vi "Auto Move Straight.vi"(7 "Target Distance":dbl=15.0 format="%#_13g", 8 "Error In":errorcluster, 11 "Refnum's In":T1) -> (0 "Error Out":errorcluster, 3 "Refnum's Out":T1)   [LabVIEW 2016]
uses:
  <vilib>/Rock Robotics/WPI/Utilities/WPI_GetSetVariantRefNum.vi
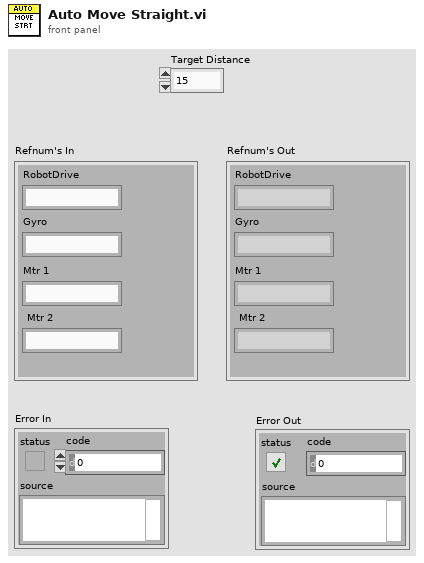
[diagram p1: front panel]
types:
  T1 = cluster{"RobotDrive":string, "Gyro":string, "Mtr 1":string, "Mtr 2":string}
  T2 = typedef "WPI_MotorControlDeviceRef.ctl" = cluster{"DeviceStatus":errorcluster, "Type":T3, "PWM":cluster{"PWM Channel":T4, "DeadBand":T5}, "CAN":cluster{"Device Number":u8, "SetOutput VI Ref":variant, "GetOutput VI Ref":variant, "Enable VI Ref":variant, "Disable VI Ref":variant, "Data":variant}, "Invert":bool}
  T3 = typedef "WPI_MotorControlType.ctl" = enum16{"PWM", "CAN"}
  T4 = typedef "FPGA_DIOPWMChannel.ctl" = enum8{"PWM 0", "PWM 1", "PWM 2", "PWM 3", "PWM 4", "PWM 5", "PWM 6", "PWM 7", "PWM 8", "PWM 9", "PWM MXP 0", "PWM MXP 1", "PWM MXP 2", "PWM MXP 3", "PWM MXP 4", "PWM MXP 5", "PWM MXP 6", "PWM MXP 7", "PWM MXP 8", "PWM MXP 9", "Invalid"}
  T5 = typedef "WPI_PWMDeadband.ctl" = cluster{"Name":string, "maxPositivePwm":i32, "minPositivePwm":i32, "centerPwm":i32, "maxNegativePwm":i32, "minNegativePwm":i32, "angularRange":u16}
  T6 = typedef "WPI_GyroDevRef.ctl" = cluster{"DevStatus":errorcluster, "Analog Channel":T7, "Offset":dbl, "Gain (VoltsPerDegree/Second)":dbl, "Gyro Type":enum16{"Analog", "XRS450"}, "Handle":i32, "SPI Bus":T8, "Device Found":bool, "Sample Rate":dbl, "Calibrate On Open":bool}
  T7 = typedef "FPGA_AIChannel.ctl" = enum8{"AI 0", "AI 1", "AI 2", "AI 3", "AI MXP 0", "AI MXP 1", "AI MXP 2", "AI MXP 3", "Invalid"}
  T8 = typedef "spi_bus.ctl" = enum16{"SPI On-Board, CS0", "SPI On-Board, CS1", "SPI On-Board, CS2", "SPI On-Board, CS3", "SPI MXP", "Invalid"}
  T9 = typedef "WPI_RobotDriveDevRef.ctl" = cluster{"DevStatus":errorcluster, "Motors[]":T2[], "Square Inputs":bool, "Max Output":dbl}
  T10 = typedef "WPI_CANTalonSRX_GlobalStatus.ctl" = cluster{"Applied Throttle":dbl, "Module Enabled":bool, "CAN Error":errorcluster, "Closed Loop Error":dbl, "Forward Limit Switch Closed":bool, "Reverse Limit Switch Closed":bool, "Sensor Position":dbl, "Sensor Velocity":dbl, "Current":dbl, "Sticky Fault - Over Temp":bool, "Sticky Fault - Under Voltage":bool, "Sticky Fault - Forward Limit":bool, "Sticky Fault - Reverse Limit":bool, "Sticky Fault - Forward Soft Limit":bool, "Sticky Fault - Reverse Soft Limit":bool, "Brake is Enabled":bool, "Encoder Position":dbl, "Encoder Velocity":dbl, "Encoder Index Count":dbl, "Encoder A Pin State":bool, "Encoder B Pin State":bool, "Encoder Index Pin State":bool, "Analog In":dbl, "Analog In Velocity":dbl, "Temperature (C)":dbl, "Battery Voltage":dbl, "Control 5 Is Supported":bool, "Current Profile Slot Select":dbl, "Pos Div 8":bool, "Vel Div 4":bool, "Pulse Width Position":i32, "Pulse Width Velocity":i32, "Pulse Width Rise To Rise (us)":i32, "Pulse Width Rise To Fall (us)":i32, "Mot Prof Active Is Under Run":bool, "Mot Prof Active Has Under Run":bool, "Mot Prof Active Is Last":bool, "Mot Prof Active Velocity Only":bool, "Mot Prof Active Is Valid":bool, "Mot Prof Buffer Is Full":bool, "Mot Prof Active Profile Slot Select":i32, "Mot Prof NextID":i32, "Mot Prof Count":i32, "Mot Prof Active Velocity":dbl, "Mot Prof Active Position":dbl, "Mot Prof Output Enable":i32}
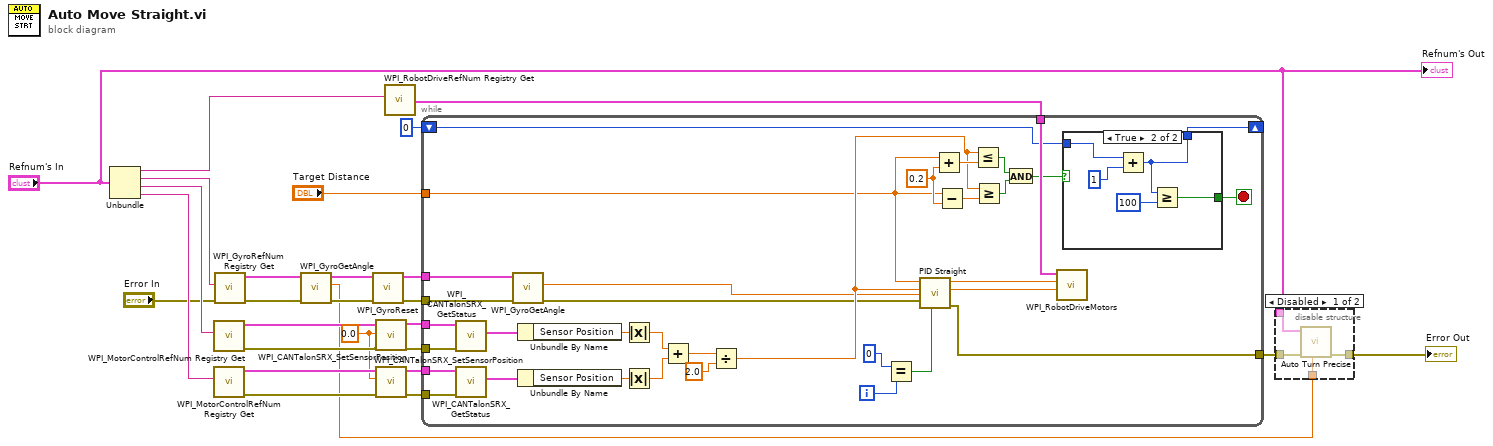
[diagram p0: block diagram]
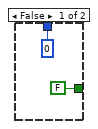
[diagram p3: hidden frame]
diagram:
  w16 = 0.0 ("New Sensor Position")
  n1 = Unbundle("Refnum's In") -> ("RobotDrive"=w11:string, "Gyro"=w10:string, "Mtr 1"=w9:string, "Mtr 2"=w8:string)
  n2 = call <vilib>:"WPI_MotorControlRefNum Registry Get.vi"("refnum name"=w9) -> ("error out"=w19:errorcluster, "MotorControlDevRef"=w20:T2)  [unwired: 9 in]
  n3 = call <vilib>:"WPI_MotorControlRefNum Registry Get.vi"("refnum name"=w8) -> ("error out"=w22:errorcluster, "MotorControlDevRef"=w21:T2)  [unwired: 9 in]
  n4 = call <vilib>:"WPI_GyroRefNum Registry Get.vi"("error in (no error)"="Error In", "refnum name"=w10) -> ("error out"=w1:errorcluster, "GyroDevRef"=w2:T6)  [unwired: 8 in]
  n5 = call <vilib>:"WPI_GyroGetAngle.vi"("error in"=w1, "GyroDevRef"=w2) -> ("error out"=w25:errorcluster, "Angle"=w3:dbl, "GyroDevRef"=w26:T6)  [unwired: 5 in, 2 out]
  n6 = call <vilib>:"WPI_GyroReset.vi"("error in"=w25, "GyroDevRef"=w26) -> ("error out"=w24:errorcluster, "GyroDevRef"=w23:T6)  [unwired: 8 in]
  n7 = call <vilib>:"WPI_CANTalonSRX_SetSensorPosition.vi"("error in (no error)"=w19, "New Sensor Position"=w16, "CAN Talon SRX Ref"=w20) -> ("error out"=w15:errorcluster, "CAN Talon SRX Ref"=w14:T2)  [unwired: 7 in]
  n8 = call <vilib>:"WPI_CANTalonSRX_SetSensorPosition.vi"("error in (no error)"=w22, "New Sensor Position"=w16, "CAN Talon SRX Ref"=w21) -> ("error out"=w17:errorcluster, "CAN Talon SRX Ref"=w18:T2)  [unwired: 7 in]
  n9 = call <vilib>:"WPI_RobotDriveRefNum Registry Get.vi"("refnum name"=w11) -> ("RobotDriveDevRef"=w12:T9)  [unwired: 9 in, 1 out]
  n10 = while {
    tunnel: w12 -> [w57]
    tunnel: w23 -> [w48]
    tunnel: w24 -> [w47]
    tunnel: w14 -> [w46]
    tunnel: w15 -> [w45]
    tunnel: w18 -> [w44]
    tunnel: w17 -> [w43]
    shift-right: [w35] -> _
    shift-left: 0 -> [w34]
    tunnel: "Target Distance" -> [w32]
    tunnel: [w29] -> w7
    i -> [w59]
    stop <- w28 stop-if-true
    w42 = 0.2 ("y")
    n11 = call <vilib>:"WPI_CANTalonSRX_GetStatus.vi"("error in (no error)"=w45, "CAN Talon SRX Ref"=w46) -> ("Talon SRX Status"=w49:T10)  [unwired: 7 in, 2 out]
    n12 = call <vilib>:"WPI_CANTalonSRX_GetStatus.vi"("error in (no error)"=w43, "CAN Talon SRX Ref"=w44) -> ("Talon SRX Status"=w50:T10)  [unwired: 7 in, 2 out]
    n13 = call <vilib>:"WPI_GyroGetAngle.vi"("error in"=w47, "GyroDevRef"=w48) -> ("error out"=w30:errorcluster, "Angle"=w33:dbl)  [unwired: 5 in, 3 out]
    n14 = Unbundle By Name(w49) -> ("Sensor Position"=w54:dbl)
    n15 = Unbundle By Name(w50) -> ("Sensor Position"=w56:dbl)
    n16 = Absolute Value(x=w54) -> (abs(x)=w53:dbl)
    n17 = Absolute Value(x=w56) -> (abs(x)=w55:dbl)
    n18 = Add(x=w53, y=w55) -> (x+y=w51:dbl)
    n19 = Divide(x=w51, y=2.0) -> (x/y=w40:dbl)
    n20 = Equal?(x=0, y=w59) -> (x = y?=w31:bool)
    n21 = call "PID Straight.vi"("Reinitialize"=w31, "Error In"=w30, "Gyro Angle"=w33, "Current Distance"=w40, "Target Distance"=w32) -> ("Error Out"=w29:errorcluster, "Right Power"=w60:dbl, "Left Power"=w61:dbl)  [unwired: 4 in]
    n22 = Add(x=w32, y=w42) -> (x+y=w41:dbl)
    n23 = Subtract(x=w32, y=w42) -> (x-y=w39:dbl)
    n24 = Less Or Equal?(x=w40, y=w41) -> (x <= y?=w38:bool)
    n25 = Greater Or Equal?(x=w40, y=w39) -> (x >= y?=w37:bool)
    n26 = And(x=w38, y=w37) -> (x .and. y?=w36:bool)
    n27 = call <vilib>:"WPI_RobotDriveMotors.vi"("RightSpeed"=w60, "LeftSpeed"=w61, "RobotDriveDevRef"=w57) -> ()  [unwired: 6 in, 3 out]
    n28 = case shown="True" w36 {
      tunnel: w34 -> [_ w67]
      tunnel: [0 w66] -> w35
      tunnel: [FALSE w64] -> w28
      frame False {
      }
      frame True {
        n29 = Add(x=w67, y=1) -> (x+y=w66:i32)
        n30 = Greater Or Equal?(x=w66, y=100) -> (x >= y?=w64:bool)
      }
    }
  }
  n31 = disable-structure shown="Disabled" {
    disable-tunnel: w7 -> [w72 _]
    disable-tunnel: [w71 _] -> w5
    disable-tunnel: "Refnum's In" -> [w70 _]
    disable-tunnel: w3 -> [w69 _]
    frame Disabled {
      n32 = call "Auto Turn Precise.vi"("Target Distance"=w69, "Error In"=w72, "Refnum's In"=w70) -> ("Error Out"=w71:errorcluster)  [unwired: 7 in, 1 out]
    }
    frame Enabled {
    }
  }
  "Error Out" <- w5
  "Refnum's Out" <- "Refnum's In"
